vi "Read Configuration.vi"(8 "error in (no error)":errorcluster, 11 "Composed Column in":refnum<class "Composed Column.lvclass">) -> (0 "error out":errorcluster, 2 "Column Interfaces.lvlib:Column Configuration.lvclass":refnum<class "Column Configuration.lvclass">, 3 "Composed Column out":refnum<class "Composed Column.lvclass">)   [LabVIEW 2020, in "Composed Columns.lvlib" / "Composed Column.lvclass"]
uses:
  Composed Column.lvclass
  Basic Columns/Column Configuration/Basic Column Configuration Class/Column Configuration.lvclass
  Composed Column.lvclass/Composed Column.ctl
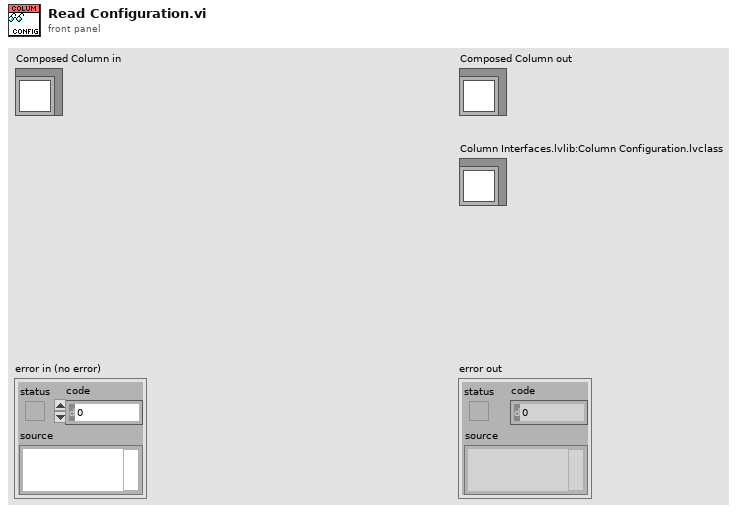
[diagram p1: front panel]
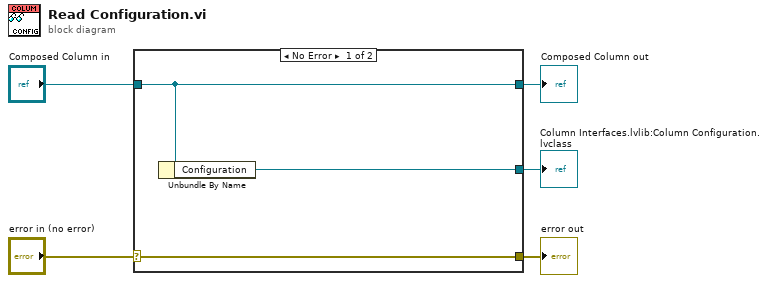
[diagram p0: block diagram]
diagram:
  n1 = case shown="No Error" "error in (no error)" {
    selector: "error in (no error)" -> [w8 w9]
    tunnel: [w8 w9] -> w4
    tunnel: [w7 w10] -> w2
    tunnel: "Composed Column in" -> [w7 w10]
    tunnel: [w6 _] -> w1
    frame No Error {
      n2 = Unbundle By Name(w7) -> ("Configuration"=w6:refnum<class "Column Configuration.lvclass">)
    }
    frame Error {
    }
  }
  "error out" <- w4
  "Composed Column out" <- w2
  "Column Interfaces.lvlib:Column Configuration.lvclass" <- w1
